vi "Sqlite Connect.vi"(5 "SqlMapper Type":refnum<class "SqlMapper.lvclass">, 6 "QuotesOnTableName":bool, 8 "error in (no error)":errorcluster, 10 "Connection String":string) -> (0 "error out":errorcluster, 3 "SqlMapper out":refnum<class "SqlMapper.lvclass">)   [LabVIEW 2020, in "ORM_DBC_Sqlite.lvlib" / "DBC.lvclass"]
uses:
  DBC.lvclass
  <vilib>/Viviota/shared/ORM.lvlibp/ORM/SqlMapper/SqlMapper.lvclass
  DBC.lvclass/DBC.ctl
  C:/Program Files/National Instruments/LabVIEW 2020/vi.lib/Viviota/shared/ORM.lvlibp/ORM/DbConnection/DbConnection.lvclass
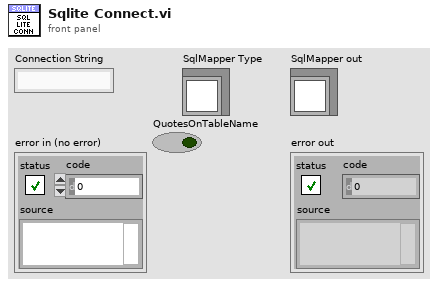
[diagram p1: front panel]
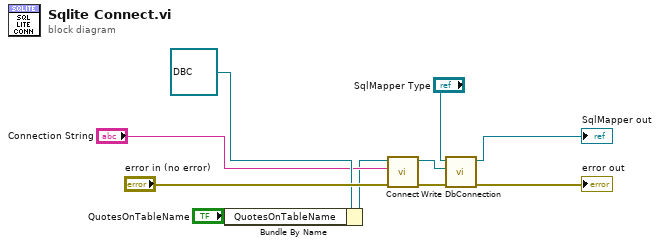
[diagram p0: block diagram]
diagram:
  n1 = Bundle By Name(cluster=refnum<class "DBC.lvclass"> refnum ("SqliteConnection in"), "QuotesOnTableName"="QuotesOnTableName") -> (w2:refnum<class "DBC.lvclass">)
  n2 = call-dynamic "Connect.vi"("error in (no error)"="error in (no error)", "Connection String"="Connection String", "SqliteConnection in"=w2) -> ("error out"=w8:errorcluster, "SqliteConnection out"=w10:refnum<class "DBC.lvclass">)  [unwired: 7 in]
  n3 = call <vilib>:"Write DbConnection.vi"("error in (no error)"=w8, "Dapper.lvlib:DbConnection.lvclass"=w10, "SqlMapper in"="SqlMapper Type") -> ("error out"=→"error out":errorcluster, "SqlMapper out"=→"SqlMapper out":refnum<class "SqlMapper.lvclass">)  [unwired: 7 in]
